vi "Increment Late Count.vi"(8 "error in (no error)":errorcluster, 11 "Transfer Group in":refnum<class "Transfer Group.lvclass">) -> (0 "error out":errorcluster, 3 "Transfer Group out":refnum<class "Transfer Group.lvclass">)   [LabVIEW 2019, in "DSF Core.lvlib" / "Transfer Group.lvclass"]
uses:
  Transfer Group.lvclass
  Transfer Group.lvclass/Transfer Group.ctl
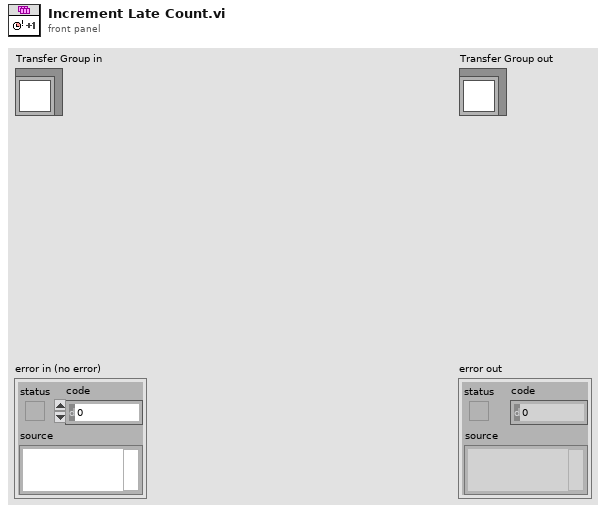
[diagram p1: front panel]
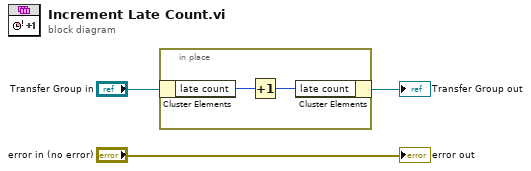
[diagram p0: block diagram]
diagram:
  n1 = in-place {
    n2 = in-place-cluster #1("Transfer Group in") -> ("late count"=w5:i32)
    n3 = Increment(x=w5) -> (x+1=w4:i32)
    n4 = in-place-cluster #1("late count"=w4) -> (→"Transfer Group out":refnum<class "Transfer Group.lvclass">)
  }
  "error out" <- "error in (no error)"
